vi "FG Current JAUS Status.vi"(1 "FG Action (Read)":T1, 2 "Status in":u8(ring)=2 items=["INIT", "READY", "STANDBY", "SHUTDOWN", "FAILURE", "EMERGENCY"]) -> (0 "Status out":u8(ring)=2 items=["INIT", "READY", "STANDBY", "SHUTDOWN", "FAILURE", "EMERGENCY"])   [LabVIEW 2011]
uses:
  cRIO/Functional Global Variables/Actions for FG's.ctl
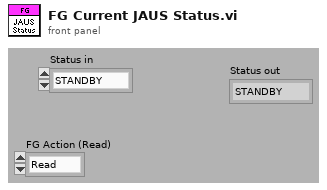
[diagram p1: front panel]
types:
  T1 = typedef "Actions for FG's.ctl" = enum16{"Read", "Write"}
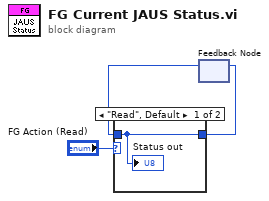
[diagram p0: block diagram]
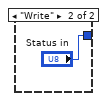
[diagram p2: hidden frame]
diagram:
  n1 = feedback #1() -> (w1:u8)  [unwired: 1 in]
  n2 = case shown="\"Read\", Default" "FG Action (Read)" {
    tunnel: w1 -> [w4 _]
    tunnel: [w4 "Status in"] -> w2
    frame "Read", Default {
      "Status out" <- w4
    }
    frame "Write" {
    }
  }
  n3 = feedback-in #1(w2) -> ()
